vi "Pre Launch Init.vi"(11 "BoundViewManager in":refnum<class "BoundViewManager.lvclass">) -> (0 "error out":errorcluster, 3 "BoundViewManager out":refnum<class "BoundViewManager.lvclass">)   [LabVIEW 2020, in "BoundViewManager.lvlib" / "BoundViewManager.lvclass"]
doc: "(<B>Filename</B>: Actor Framework.lvlib:Actor.lvclass:Pre Launch Init.vi)\n\nDefines behavior that occurs after the Launch Nested Actor method is invoked but before the actor's Actor Core method begins running.\n\nBy default, this method does nothing. A descendant class may override it to define behavior.\n\n<License>\nCopyright © 2017 Composed Systems, LLC | All rights reserved\nwww.composed.io\n\nAuthor: Ethan Stern <ethan.stern@composed.io>\n\nThis software is provided \"AS IS\" WITHOUT WARRANTIES, either express or implied, AND IS FOR EDUCATIONAL PURPOSES ONLY.\n</License>"
uses:
  BoundViewManager.lvclass
  BoundViewManager.lvclass/BoundViewManager.ctl
  modules/mva-core/Source/IObserver/IObserver/IObserver.lvclass
  modules/mva-core/Source/SubscriptionPolicy/ValueChangeSubscription/ValueChangeSubscription.lvclass
  modules/mva-core/Source/SubscriptionPolicy/BasicSubscription/BasicSubscription.lvclass
  modules/composed-lookup-table/Source/LookupTable/LookupTable.lvclass
  modules/mva-viewable/Source/IViewManager/IViewManager/IViewManager.lvclass
  BoundViewManager Messages/Insert Bound View Msg/Insert Bound View Msg.lvclass
  C:/Program Files/National Instruments/LabVIEW 2020/vi.lib/ActorFramework/Message/Message.lvclass
  C:/Program Files/National Instruments/LabVIEW 2020/vi.lib/ActorFramework/Actor/Actor.lvclass
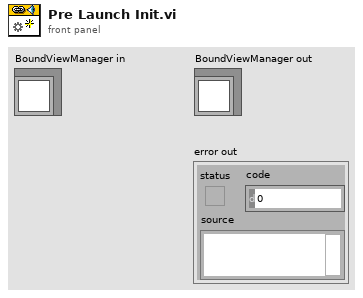
[diagram p1: front panel]
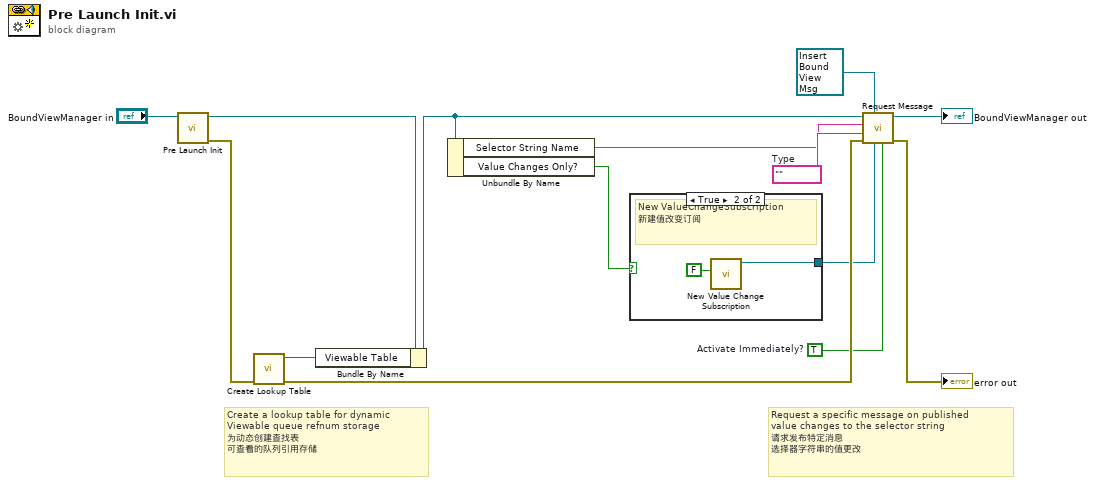
[diagram p0: block diagram]
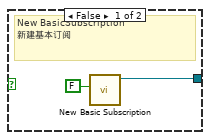
[diagram p2: hidden frame]
diagram:
  w4 = TRUE  # Activate Immediately?
  w7 = ""  # Type
  # "Request a specific message on published\nvalue changes to the selector string\n请求发布特定消息\n选择器字符串的值更改"
  # "Create a lookup table for dynamic\nViewable queue refnum storage\n为动态创建查找表\n可查看的队列引用存储"
  n1 = call-parent "Pre Launch Init.vi"("IViewManager in"="BoundViewManager in") -> ("error out"=w12:errorcluster, "IViewManager out"=w14:refnum<class "BoundViewManager.lvclass">)  [unwired: 9 in]
  n2 = call "Create Lookup Table.vi"("error in (no error)"=w12) -> ("error out"=w9:errorcluster, "LookupTable Reference"=w11:refnum<data-value>)  [unwired: 9 in]
  n3 = Bundle By Name(cluster=w14, "Viewable Table"=w11) -> (w6:refnum<class "BoundViewManager.lvclass">)
  n4 = Unbundle By Name(w6) -> ("Selector String Name"=w5:string, "Value Changes Only?"=w3:bool)
  n5 = case shown="True" w3 {
    tunnel: [w16 w18] -> w2
    frame False {
      # "New BasicSubscription\n新建基本订阅"
      n6 = call "New Basic Subscription.vi"("Ignore Past Updates? (F)"=FALSE) -> ("BasicSubscription Out"=w16:refnum<class "BasicSubscription.lvclass">)  [unwired: 10 in]
    }
    frame True {
      # "New ValueChangeSubscription\n新建值改变订阅"
      n7 = call "New Value Change Subscription.vi"("Ignore Past Updates? (F)"=FALSE) -> ("ValueChangeSubscription Out"=w18:refnum<class "ValueChangeSubscription.lvclass">)  [unwired: 10 in]
    }
  }
  n8 = call "Request Message.vi"("Activate Immediately? (T)"=w4, "Configured SubscriptionPolicy"=w2, "Desired Notification Msg"=refnum<class "Insert Bound View Msg.lvclass"> refnum ("BoundViewManager.lvlib:Insert Bound View Msg.lvclass"), "error in (no error)"=w9, "Data Type"=w7, "Datum Name"=w5, "IObserver in"=w6) -> ("error out"=→"error out":errorcluster, "IObserver in"=→"BoundViewManager out":refnum<class "BoundViewManager.lvclass">)  [unwired: 2 in, 1 out]
